vi "Write Panel Ref 1.vi"(8 "error in (no error)":errorcluster, 10 "Panel Ref":refnum<vi>, 11 "Abstruct View in":refnum<class "Abstruct View.lvclass">) -> (0 "error out":errorcluster, 3 "Abstruct View out":refnum<class "Abstruct View.lvclass">)   [LabVIEW 2020, in "Abstruct View.lvlib" / "Abstruct View.lvclass"]
uses:
  Abstruct View.lvclass
  Abstruct View.lvclass/Abstruct View.ctl
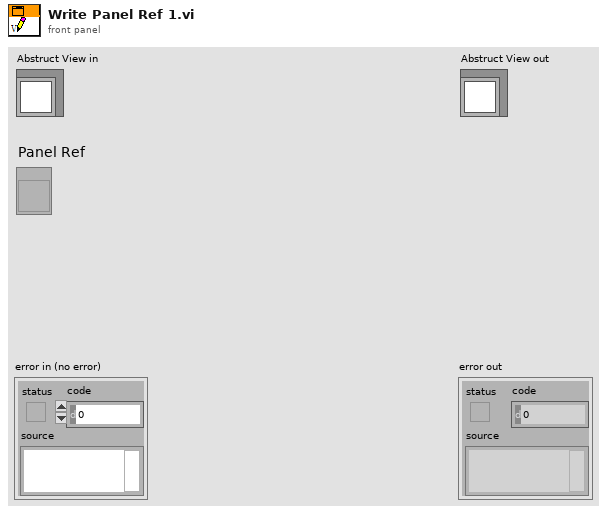
[diagram p1: front panel]
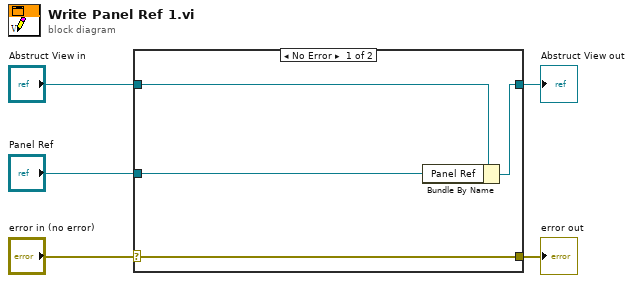
[diagram p0: block diagram]
diagram:
  n1 = case shown="No Error" "error in (no error)" {
    selector: "error in (no error)" -> [w9 w10]
    tunnel: [w9 w10] -> w4
    tunnel: [w7 w11] -> w2
    tunnel: "Abstruct View in" -> [w8 w11]
    tunnel: "Panel Ref" -> [w6 _]
    frame No Error {
      n2 = Bundle By Name(cluster=w8, "Panel Ref"=w6) -> (w7:refnum<class "Abstruct View.lvclass">)
    }
    frame Error {
    }
  }
  "error out" <- w4
  "Abstruct View out" <- w2
